vi "countTestCases.vi"(8 "error in (no error)":errorcluster, 11 "TestSuite in":refnum<class "TestSuite.lvclass">) -> (0 "error out":errorcluster, 2 "count":u32, 3 "TestSuite out":refnum<class "TestSuite.lvclass">)   [LabVIEW 2019, in "TestSuite.lvclass"]
uses:
  TestSuite.lvclass
  TestSuite.lvclass/TestSuite.ctl
  TestCase/TestCase.lvclass
panel:
  # "JKI VI Tester for LabVIEW\nhttp://jkisoft.com/vi-tester\nCopyright (C) 2007-2009, JKI <info@jkisoft.com>\nALL RIGHTS RESERVED"
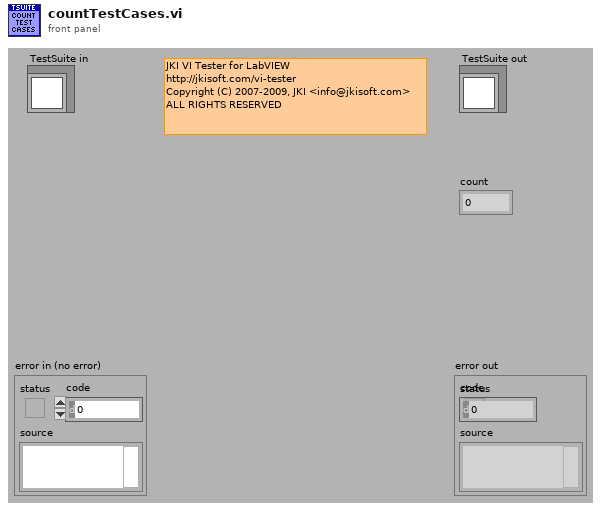
[diagram p1: front panel]
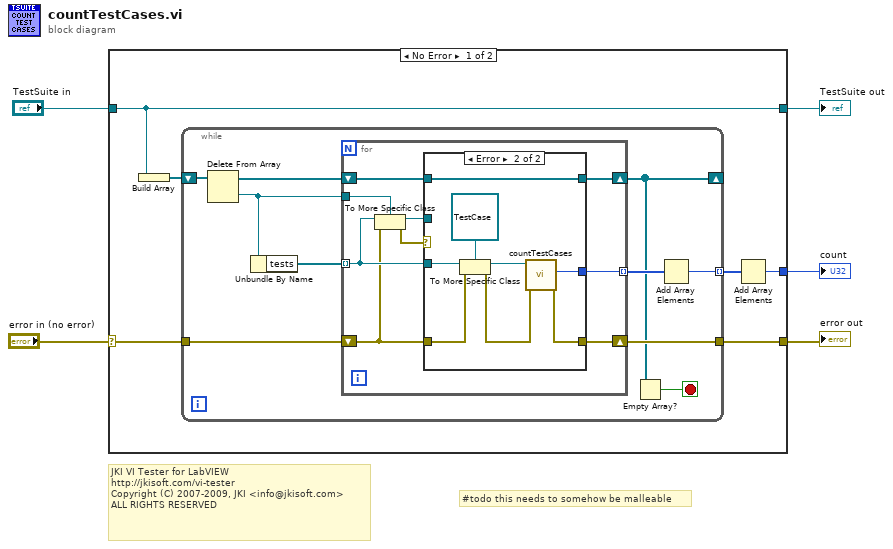
[diagram p0: block diagram]
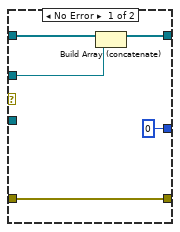
[diagram p2: hidden frame]
diagram:
  # "#todo this needs to somehow be malleable"
  # "JKI VI Tester for LabVIEW\nhttp://jkisoft.com/vi-tester\nCopyright (C) 2007-2009, JKI <info@jkisoft.com>\nALL RIGHTS RESERVED"
  n1 = case shown="No Error" "error in (no error)" {
    selector: "error in (no error)" -> [w11 w45]
    tunnel: [w10 w45] -> w4
    tunnel: [w9 w44] -> w2
    tunnel: "TestSuite in" -> [w9 w44]
    tunnel: [w6 _] -> w1
    frame No Error {
      n2 = Build Array(w9) -> (w8:refnum<class "TestSuite.lvclass">[])
      n3 = while {
        tunnel: w11 -> [w20]
        tunnel: [w19] -> w10
        shift-right: [w13] -> _
        shift-left: w8 -> [w17]
        tunnel: [w12] -> w7 mode=indexing
        stop <- w14 stop-if-true
        n4 = Delete From Array(array=w17) -> (deleted portion=w16:refnum<class "TestSuite.lvclass">, array with subset deleted=w15:refnum<class "TestSuite.lvclass">[])  [unwired: 2 in]
        n5 = Unbundle By Name(w16) -> ("tests"=w21:refnum<class>[])
        n6 = for {
          tunnel: w21 -> [w27] mode=indexing
          tunnel: [w30] -> w18 mode=indexing
          shift-right: [w29] -> w19
          shift-left: w20 -> [w25]
          tunnel: w16 -> [w28]
          shift-right: [w24] -> w13
          shift-left: w15 -> [w23]
          n7 = To More Specific Class(target class=w28, reference=w27, error in=w25) -> (specific class reference=w22:refnum<class "TestSuite.lvclass">, error out=w26:errorcluster)
          n8 = case shown="Error" w26 {
            tunnel: [u32 0 ("count") w41] -> w30
            tunnel: [w31 w39] -> w29
            tunnel: w27 -> [_ w38]
            tunnel: w25 -> [w31 w37]
            tunnel: [w33 w36] -> w24
            tunnel: w23 -> [w34 w36]
            tunnel: w22 -> [w35 _]
            frame No Error {
              n9 = Build Array (concatenate)(w34, w35) -> (w33:refnum<class "TestSuite.lvclass">[])
            }
            frame Error {
              n10 = To More Specific Class(target class=refnum<class "TestCase.lvclass"> refnum ("reference in"), reference=w38, error in=w37) -> (specific class reference=w42:refnum<class "TestCase.lvclass">, error out=w40:errorcluster)
              n11 = call-dynamic "countTestCases.vi"("error in (no error)"=w40, "TestCase in"=w42) -> ("error out"=w39:errorcluster, "count"=w41:u32)  [unwired: 7 in, 1 out]
            }
          }
        }
        n12 = Empty Array?(array=w13) -> (empty?=w14:bool)
        n13 = Add Array Elements(numeric array=w18) -> (sum=w12:u32)
      }
      n14 = Add Array Elements(numeric array=w7) -> (sum=w6:u32)
    }
    frame Error {
    }
  }
  "error out" <- w4
  "TestSuite out" <- w2
  "count" <- w1
